vi "ADS1015 Read All.vi"(7 "I2C Channel":u8, 8 "error in (no error)":errorcluster, 9 "ADS1015 Config Options":T1={"Channel"=4, "Expected Range (Programmable Gain Amplifier)"=0, "Sampling Mode"=1, "Sampling Rate"=4, "Comparator Mode"=1, "Comparator Polarity"=1, "Latching Comparator"=1, "Comparator Queue & Disable"=3} {"Comparator Queue & Disable" items=["Assert after one conversion", "Assert after two conversions", "Assert after four conversions", "Comparator disabled"]; "Latching Comparator" items=["Non-latching", "Latching"]; "Comparator Polarity" items=["Active Low", "Active High"]; "Comparator Mode" items=["Traditional Comparator w/ hysteresis", "Window Comparator"]; "Sampling Rate" items=["128SPS", "250SPS", "490SPS", "920SPS", "1600SPS", "2400SPS", "3300SPS"]; "Sampling Mode" items=["Continuous Conversion", "Single-shot (Low Power)"]; "Expected Range (Programmable Gain Amplifier)" items=["+/-6.144V", "+/-4.096V", "+/-2.048V", "+/-1.024V", "+/-0.512V", "+/-0.256V"]; "Channel" items=["Differential: Ch 0&1", "Differential: Ch 0&3", "Differential: Ch 1&3", "Differential: Ch 2&3", "Single Ended: Ch 0", "Single Ended: Ch 1", "Single Ended: Ch 2", "Single Ended: Ch 3"]}, 10 "I2C Slave Address":u8 format="%.0x", 11 "LINX Resource in":T2) -> (0 "error out":errorcluster, 2 "Voltages":dbl[](array[numeric]) format="%.3f V", 3 "LINX Resource":T2, 4 "Resolution":dbl format="%.3f V")   [LabVIEW 2014]
uses:
  <vilib>/MakerHub/LINX/Private/Type Defs/LINX Ref.ctl
  <vilib>/MakerHub/LINX/Private/Type Defs/Platform.ctl
  <vilib>/MakerHub/LINX/Private/Type Defs/Interface.ctl
  <vilib>/MakerHub/LINX/Private/Device/Type Defs/LINX Device Config.ctl
  <vilib>/MakerHub/LINX/Private/Device/Type Defs/TCP Config.ctl
  <vilib>/MakerHub/LINX/Private/Device/Type Defs/Channels.ctl
  ADS1015 Config Options.ctl
  <vilib>/MakerHub/LINX/Private/Local IO/LinxI2cWrite.vi
  <vilib>/MakerHub/LINX/Public/Utilities/Check Channel.vi
  <vilib>/myRIO/Instrument Drivers/Onboard IO/I2C/vis/Write.vi
  <vilib>/MakerHub/LINX/Private/Utilties/Generate Error.vi
  <vilib>/MakerHub/LINX/Private/Utilties/Channel FGVs/I2C Channels.vi
  <vilib>/Utility/error.llb/Error Cluster From Error Code.vi
  <vilib>/myRIO/Common/Instrument Driver Framework/myRIO v1.0/I2C/vis/myRIO v1.0 Write I2C.vi
  <vilib>/MakerHub/LINX/LMH-LINX.lvlib
  <vilib>/MakerHub/LINX/Private/Device/Device.lvlib
panel:
  out "Raw Reading":u16 format="%.0x"
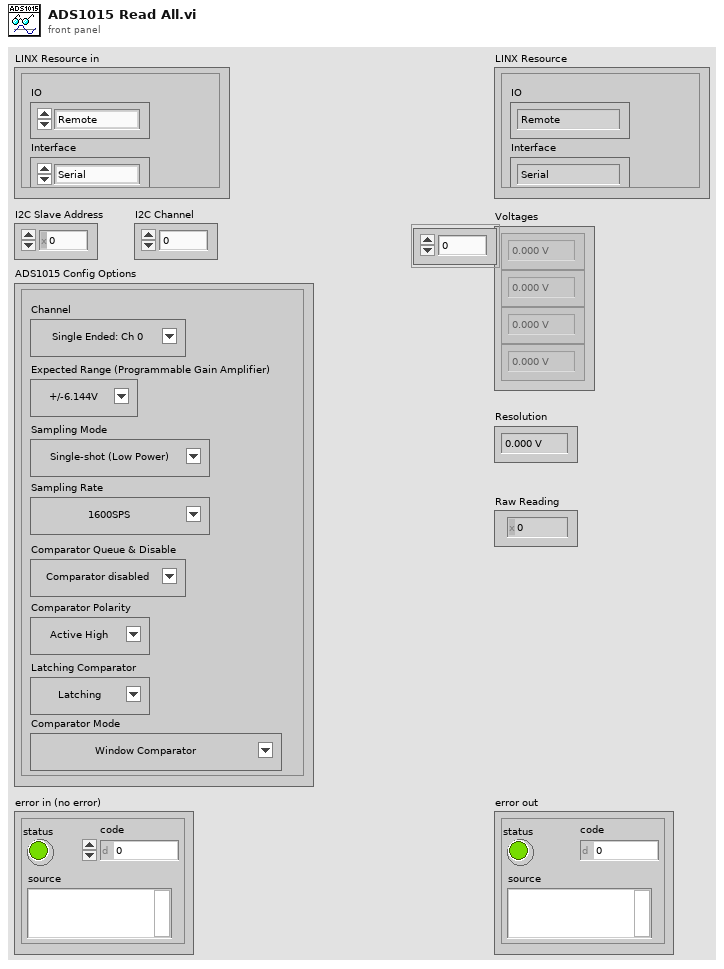
[diagram p1: front panel]
types:
  T1 = typedef "ADS1015 Config Options.ctl" = cluster{"Channel":u8, "Expected Range (Programmable Gain Amplifier)":u8, "Sampling Mode":u8, "Sampling Rate":u8, "Comparator Mode":u8, "Comparator Polarity":u8, "Latching Comparator":u8, "Comparator Queue & Disable":u8}
  T2 = typedef "LMH-LINX.lvlib/LINX Ref.ctl" = cluster{"IO":T3, "Interface":T4, "LINX Device Config":T5}
  T3 = typedef "LMH-LINX.lvlib/Platform.ctl" = enum16{"Remote", "Local"}
  T4 = typedef "LMH-LINX.lvlib/Interface.ctl" = enum16{"Serial", "TCP"}
  T5 = typedef "LMH-LINX.lvlib/Device.lvlib/LINX Device Config.ctl" = cluster{"Interface":T4, "COM Port":refnum<visa-resource-name>, "TCP Configuration":T6, "Device Family":u8, "Device ID":u8, "Device Name":string, "TCP Ref":refnum<k5>, "Channels":T7}
  T6 = typedef "LMH-LINX.lvlib/Device.lvlib/TCP Config.ctl" = cluster{"IP Address":string, "Port":u16}
  T7 = typedef "LMH-LINX.lvlib/Channels.ctl" = cluster{"DI":u8[], "DO":u8[], "AI":u8[], "AO":u8[], "PWM":u8[], "QE":u8[], "UART":u8[], "I2C 2":u8[], "SPI":u8[], "CAN":u8[], "Servo":u8[], "AI Ref (V)":dbl, "AI Resolution (Bits)":u8, "AO Ref (V)":dbl, "AO Resolution (Bits)":u8}
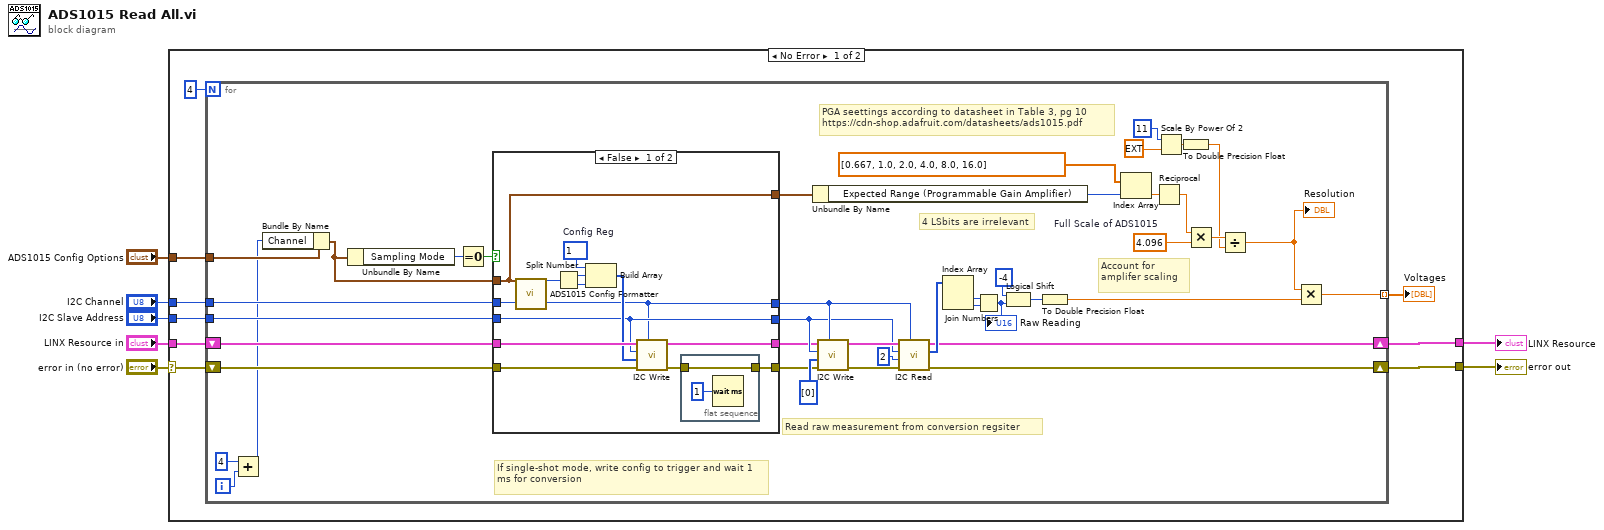
[diagram p0: block diagram]
diagram:
  n1 = case shown="No Error" "error in (no error)" {
    selector: "error in (no error)" -> [w13 w78]
    tunnel: "LINX Resource in" -> [w14 w79]
    tunnel: "I2C Channel" -> [w16 _]
    tunnel: "I2C Slave Address" -> [w15 _]
    tunnel: "ADS1015 Config Options" -> [w12 _]
    tunnel: [w11 w79] -> w2
    tunnel: [w10 w78] -> w1
    frame No Error {
      n2 = for {
        N: 4 -> [_]
        tunnel: w16 -> [w51]
        tunnel: w15 -> [w50]
        tunnel: w12 -> [w21]
        tunnel: [w28] -> w9 mode=indexing
        shift-right: [w42] -> w11
        shift-left: w14 -> [w49]
        shift-right: [w41] -> w10
        shift-left: w13 -> [w48]
        i -> [w19]
        w32 = 4.096  # Full Scale of ADS1015
        # "Account for amplifer scaling"
        # "PGA seettings according to datasheet in Table 3, pg 10\nhttps://cdn-shop.adafruit.com/datasheets/ads1015.pdf"
        # "4 LSbits are irrelevant"
        # "Read raw measurement from conversion regsiter"
        # "If single-shot mode, write config to trigger and wait 1 ms for conversion"
        n3 = Add(x=4, y=w19) -> (x+y=w17:i32)
        n4 = Bundle By Name(cluster=w21, "Channel"=w17) -> (w20:T1)
        n5 = Unbundle By Name(w20) -> ("Sampling Mode"=w53:u8)
        n6 = Equal To 0?(x=w53) -> (x = 0?=w52:bool)
        n7 = case shown="False" w52 {
          tunnel: w51 -> [w61 w77]
          tunnel: w50 -> [w62 w76]
          tunnel: w49 -> [w66 w75]
          tunnel: w48 -> [w65 w74]
          tunnel: [w61 w77] -> w47
          tunnel: [w62 w76] -> w46
          tunnel: [w63 w75] -> w45
          tunnel: [w58 w74] -> w44
          tunnel: w20 -> [w60 w73]
          tunnel: [w60 w73] -> w37
          frame False {
            w68 = u8 1  # Config Reg
            n8 = call "ADS1015 Config Formatter.vi"("ADS1015 Config Options"=w60) -> ("Config Command"=w67:u16)  [unwired: 10 in]
            n9 = Split Number(x=w67) -> (hi(x)=w70:u8, lo(x)=w69:u8)
            n10 = Build Array(w68, w70, w69) -> (w64:u8[])
            n11 = call <vilib>:"I2C Write.vi"("I2C Channel"=w61, "Error In"=w65, "Data"=w64, "I2C Slave Address (0)"=w62, "LINX Resource"=w66) -> ("Error Out"=w59:errorcluster, "LINX Resource"=w63:T2)  [unwired: 5 in]
            n12 = flat-sequence {
              tunnel: w59 -> [w72]
              tunnel: [w72] -> w58
              frame #0 {
                n13 = Wait (ms)(milliseconds to wait=u32 1) -> ()  [unwired: 1 out]
              }
            }
          }
          frame True {
          }
        }
        n14 = Unbundle By Name(w37) -> ("Expected Range (Programmable Gain Amplifier)"=w35:u8)
        n15 = call <vilib>:"I2C Write.vi"("I2C Channel"=w47, "Error In"=w44, "Data"=u8[] [0], "I2C Slave Address (0)"=w46, "LINX Resource"=w45) -> ("Error Out"=w56:errorcluster, "LINX Resource"=w57:T2)  [unwired: 5 in]
        n16 = call <vilib>:"I2C Read.vi"("I2C Channel"=w47, "Error In"=w56, "Bytes To Read"=u8 2, "I2C Slave Address (0)"=w46, "LINX Resource"=w57) -> ("Error Out"=w41:errorcluster, "Data"=w43:u8[], "LINX Resource"=w42:T2)  [unwired: 4 in]
        n17 = Index Array(array=w43) -> (element #1=w39:u8, element #2=w40:u8)  [unwired: 2 in]
        n18 = Join Numbers(hi=w39, lo=w40) -> ((hi.lo)=w38:u16)
        "Raw Reading" <- w38
        n19 = Logical Shift(y=i16 -4, x=w38) -> (x << y=w22:u16)
        n20 = To Double Precision Float(number=w22) -> (double precision float=w30:dbl)
        n21 = Index Array(array=dbl[] [0.667, 1.0, 2.0, 4.0, 8.0, 16.0] ("Data"), index=w35) -> (element=w33:dbl)
        n22 = Reciprocal(x=w33) -> (1/x=w31:dbl)
        n23 = Scale By Power Of 2(n=i16 11, x=ext 1.0) -> (x*2^n=w25:ext)
        n24 = To Double Precision Float(number=w25) -> (double precision float=w23:dbl)
        n25 = Multiply(x=w31, y=w32) -> (x*y=w29:dbl)
        n26 = Divide(x=w29, y=w23) -> (x/y=w27:dbl)
        "Resolution" <- w27
        n27 = Multiply(x=w27, y=w30) -> (x*y=w28:dbl)
      }
      "Voltages" <- w9
    }
    frame Error {
    }
  }
  "error out" <- w1
  "LINX Resource" <- w2
